vi "fgv_4610_config.vi"(7 "cmd":T2, 8 "error in (no error)":errorcluster, 11 "BP4610 Config":T1={"VISA"="", "Limit-BP"={"Set"=enum."Current", "Voltage+[V]"=20.0, "Current+[A]"=5.0, "Voltage-[V]"=-20.0, "Current-[A]"=-5.0}, "SET BP"={"Set"=enum."FREQ/WAVE", "Operation mode"=0, "Voltage[Vp-p]"=0.0, "Current[Ap-p]"=0.0, "Voltage[V]"=0.0, "Current[A]"=0.0, "Frequency[Hz]"=1.0, "Waveform"=enum."Sine"}} {"SET BP"."Frequency[Hz]" min=1.0 max=100000.0 step=0.1; "SET BP"."Current[A]" min=-20.0 max=20.0 step=0.001; "SET BP"."Voltage[V]" min=-115.0 max=115.0 step=0.01; "SET BP"."Current[Ap-p]" min=0.0 max=60.0 step=0.01; "SET BP"."Voltage[Vp-p]" min=0.0 max=120.0 step=0.1; "SET BP"."Operation mode" items=["CV-INT", "CV-EXT", "CV-ADD", "CC-INT", "CC-EXT", "CC-ADD"]; "Limit-BP"."Current-[A]" min=-20.0 max=20.0 step=0.001; "Limit-BP"."Voltage-[V]" min=-115.0 max=115.0 step=0.01; "Limit-BP"."Current+[A]" min=0.0 max=60.0 step=0.01; "Limit-BP"."Voltage+[V]" min=0.0 max=120.0 step=0.1}) -> (0 "error out":errorcluster, 3 "BP4610 Config 2":T1={"VISA"="", "Limit-BP"={"Set"=enum."Current", "Voltage+[V]"=20.0, "Current+[A]"=5.0, "Voltage-[V]"=-20.0, "Current-[A]"=-5.0}, "SET BP"={"Set"=enum."FREQ/WAVE", "Operation mode"=0, "Voltage[Vp-p]"=0.0, "Current[Ap-p]"=0.0, "Voltage[V]"=0.0, "Current[A]"=0.0, "Frequency[Hz]"=1.0, "Waveform"=enum."Sine"}} {"SET BP"."Frequency[Hz]" min=1.0 max=100000.0 step=0.1; "SET BP"."Current[A]" min=-20.0 max=20.0 step=0.001; "SET BP"."Voltage[V]" min=-115.0 max=115.0 step=0.01; "SET BP"."Current[Ap-p]" min=0.0 max=60.0 step=0.01; "SET BP"."Voltage[Vp-p]" min=0.0 max=120.0 step=0.1; "SET BP"."Operation mode" items=["CV-INT", "CV-EXT", "CV-ADD", "CC-INT", "CC-EXT", "CC-ADD"]; "Limit-BP"."Current-[A]" min=-20.0 max=20.0 step=0.001; "Limit-BP"."Voltage-[V]" min=-115.0 max=115.0 step=0.01; "Limit-BP"."Current+[A]" min=0.0 max=60.0 step=0.01; "Limit-BP"."Voltage+[V]" min=0.0 max=120.0 step=0.1})   [LabVIEW 2019]
uses:
  _ctrl/rw.ctl
  _ctrl/BP4610_config.ctl
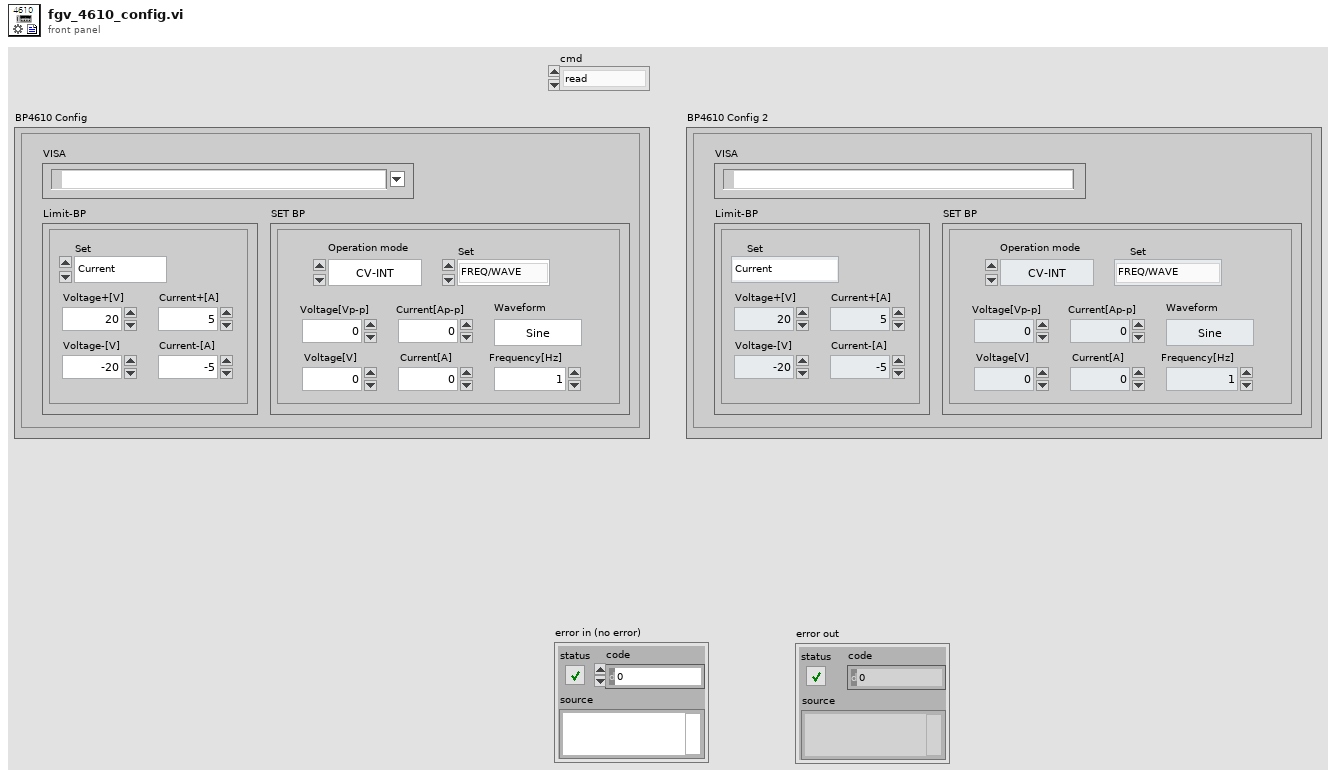
[diagram p1: front panel]
types:
  T1 = typedef "BP4610_config.ctl" = cluster{"VISA":refnum<visa-resource-name>, "Limit-BP":cluster{"Set":enum16{"Current", "Voltage"}, "Voltage+[V]":dbl, "Current+[A]":dbl, "Voltage-[V]":dbl, "Current-[A]":dbl}, "SET BP":cluster{"Set":enum16{"Current", "Voltage", "FREQ/WAVE"}, "Operation mode":u16, "Voltage[Vp-p]":dbl, "Current[Ap-p]":dbl, "Voltage[V]":dbl, "Current[A]":dbl, "Frequency[Hz]":dbl, "Waveform":enum16{"Sine", "Square", "ARB 1", "ARB 2", "ARB 3", "ARB 4", "ARB 5", "ARB 6", "ARB 7", "ARB 8", "ARB 9", "ARB 10", "ARB 11", "ARB 12", "ARB 13", "ARB 14", "ARB 15", "ARB 16"}}}
  T2 = typedef "rw.ctl" = enum16{"read", "write"}
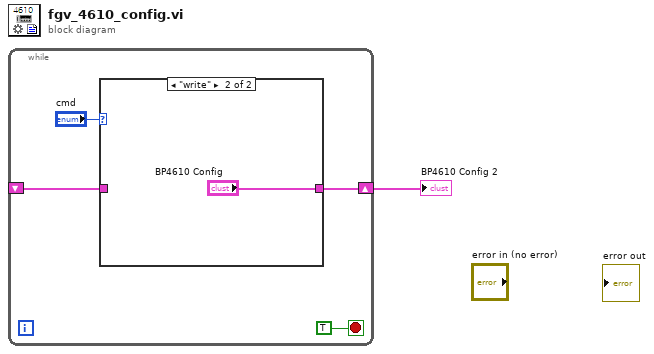
[diagram p0: block diagram]
diagram:
  n1 = while {
    shift-right: [w3] -> w1
    shift-left: _ -> [w2]
    stop <- TRUE stop-if-true
    n2 = case shown="\"write\"" "cmd" {
      tunnel: [w6 "BP4610 Config"] -> w3
      tunnel: w2 -> [w6 _]
      frame "read", Default {
      }
      frame "write" {
      }
    }
  }
  "BP4610 Config 2" <- w1
